vi "Open Device Types from File.vi"(2 "Error In":errorcluster) -> (0 "Error Out":errorcluster, 1 "Device Types":string[](array[string]))   [LabVIEW 2019]
uses:
  <vilib>/Utility/config.llb/Read Key (String).vi
  <vilib>/Utility/config.llb/NI_LVConfig.lvlib
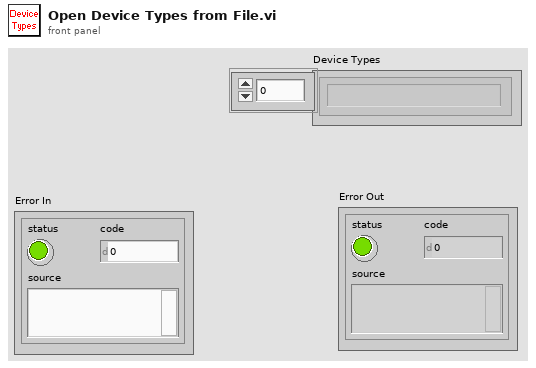
[diagram p1: front panel]
types:
  T1 = typedef "NI_LVConfig.lvlib/Config Data RefNum.ctl" = refnum<k1>
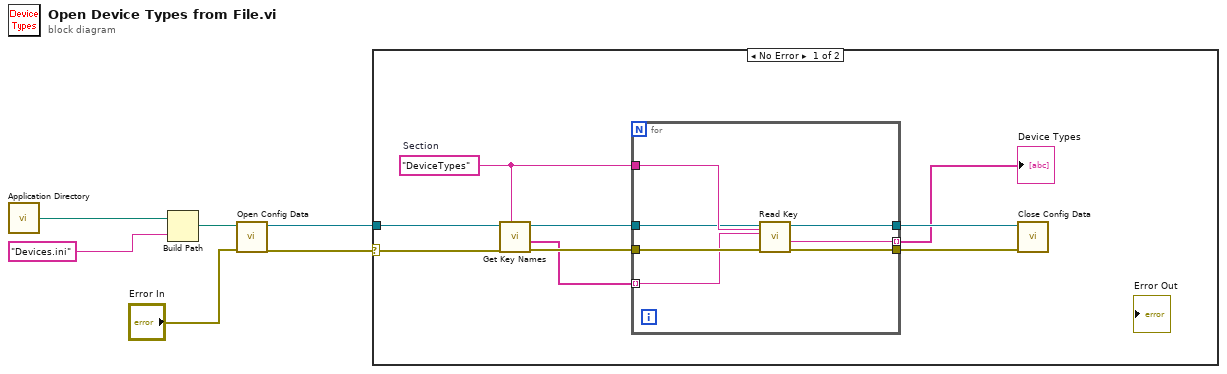
[diagram p0: block diagram]
diagram:
  n1 = call <vilib>:"Application Directory.vi"() -> ("Application Directory"=w6:path)
  n2 = Build Path(base path=w6, name or relative path="Devices.ini") -> (appended path=w4:path)
  n3 = call <vilib>:"Open Config Data.vi"("error in (no error)"="Error In", "configuration file path"=w4) -> ("error out"=w2:errorcluster, "refnum"=w3:T1)  [unwired: 7 in, 1 out]
  n4 = case shown="No Error" w2 {
    selector: w2 -> [w8 _]
    tunnel: w3 -> [w15 _]
    frame No Error {
      w14 = "DeviceTypes"  # Section
      n5 = call <vilib>:"Get Key Names.vi"("section"=w14, "error in (no error)"=w8, "refnum"=w15) -> ("error out"=w12:errorcluster, "key names"=w11:string[], "refnum out"=w13:T1)  [unwired: 5 in, 1 out]
      n6 = for {
        tunnel: w14 -> [w22]
        tunnel: w13 -> [w21]
        tunnel: w12 -> [w20]
        tunnel: w11 -> [w19] mode=indexing
        tunnel: [w18] -> w7 mode=indexing
        tunnel: [w17] -> w10
        tunnel: [w16] -> w9
        n7 = call-poly <vilib>:"Read Key.vi"("section"=w22, "error in (no error)"=w20, "key"=w19, "refnum"=w21) -> ("error out"=w16:errorcluster, "value"=w18:string, "refnum out"=w17:T1)  [unwired: 4 in, 1 out]
      }
      "Device Types" <- w7
      n8 = call <vilib>:"Close Config Data.vi"("error in (no error)"=w9, "refnum"=w10) -> ()  [unwired: 8 in, 2 out]
    }
    frame Error {
    }
  }
